vi "차선 보간(차량 가까운점).vi"(3 "Vision Theta":dbl[](array[numeric]), 4 "Vision Distance":dbl[](array[numeric]), 5 "Lane":dbl[][](array[numeric])) -> (0 "thetam":dbl[](array[numeric]), 1 "rm":dbl[](array[numeric]), 2 "Vision":dbl[][](array[numeric]))   [LabVIEW 2016]
uses:
  <vilib>/imath/engines/lvmath2/RunTimeEngine/Managers/WorkSpace/UID Generator.vi
  <vilib>/imath/engines/lvmath2/RunTimeEngine/RunTimeType/NIMS_RunTimeType_From StrictType (excl LVString).vi
  <instcachedir>/0/NIMS_RunTimeType_From StrictType (excl LVString)_BBF44FB49F834B71AF7A14CCEDF8BECD.lvgen/NIMS_RunTimeType_From StrictType (excl LVString)_BBF44FB49F834B71AF7A14CCEDF8BECD_000.vi
  <vilib>/imath/engines/lvmath2/RunTimeEngine/LocalVariableDefStatement/MC_LocalVariableDefStatement_Display.vi
  <vilib>/imath/engines/lvmath2/RunTimeEngine/MatrixToken/NIMS_MatrixToken_M_M.vi
  <instcachedir>/0/NIMS_MatrixToken_M_M_DF273B0CC20F424BBF1EDA9F4E71C841.lvgen/NIMS_MatrixToken_M_M_DF273B0CC20F424BBF1EDA9F4E71C841_003.vi
  <vilib>/imathl/engines/lvmath/Functions/Error Handling/Create Error.vi
  <vilib>/imath/engines/lvmath2/RunTimeEngine/Managers/SymbolTable/Clear UID.vi
  <vilib>/imath/engines/lvmath2/RunTimeEngine/NodeEndStatement/NIMS_NodeEndStatement_Output.vi
  <instcachedir>/0/NIMS_NodeEndStatement_Output_53EC0D466D134D7ABD903AC30B43404B.lvgen/NIMS_NodeEndStatement_Output_53EC0D466D134D7ABD903AC30B43404B_003.vi
  <instcachedir>/0/NIMS_NodeEndStatement_Output_53EC0D466D134D7ABD903AC30B43404B.lvgen/NIMS_NodeEndStatement_Output_53EC0D466D134D7ABD903AC30B43404B_000.vi
  <vilib>/imath/engines/lvmath2/RunTimeEngine/ErrorHandling/NIMS_Finalize Error.vi
  <vilib>/imath/engines/lvmath2/RunTimeEngine/Managers/SymbolTable/NIMS_WorkSpace.lvlib
panel:
  out "Xm":dbl[][](array[numeric])
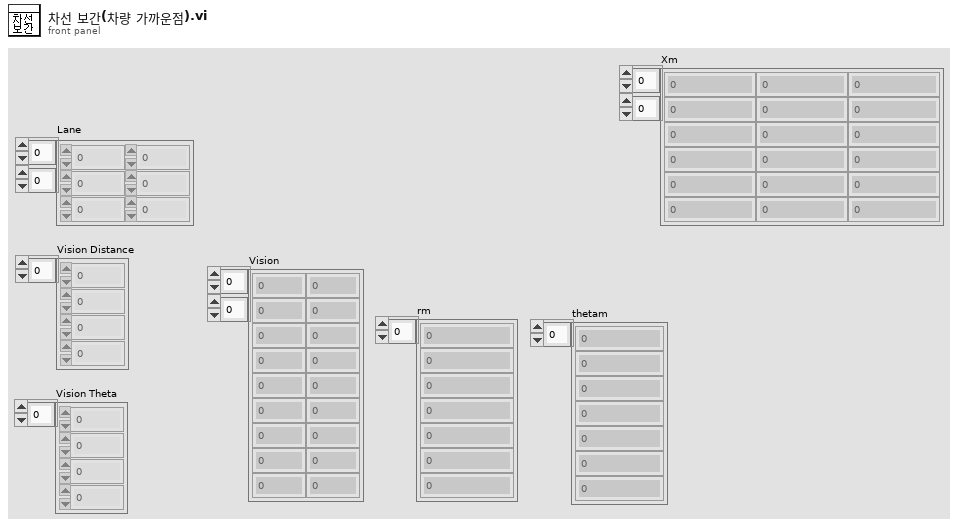
[diagram p1: front panel]
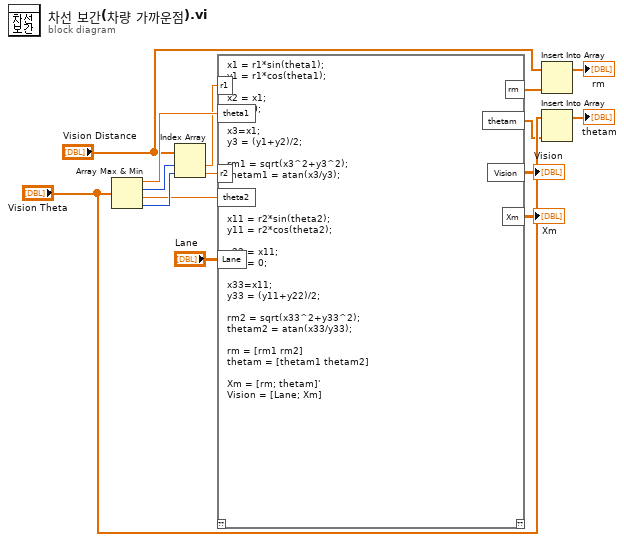
[diagram p0: block diagram]
diagram:
  n1 = Array Max & Min(array="Vision Theta") -> (max value=w13:dbl, max index (indices)=w15:i32, min value=w10:dbl, min index (indices)=w14:i32)
  n2 = Index Array(array="Vision Distance", index #1=w15, index #2=w14) -> (element #1=w12:dbl, element #2=w11:dbl)
  n3 = mathscript code="x1 = r1*sin(theta1);\ny1 = r1*cos(theta1);\n\nx2 = x1;\ny2 = 0;\n\nx3=x1;\ny3 = (y1+y2)/2;\n\nrm1 = sqrt(x3^2+y3^2);\nthetam1 = atan(x3/y3);\n\n\n\nx11 = r2*sin(theta2);\ny11 = r2*cos(theta2);\n\nx22 = x11;\ny22 = 0;\n\nx33=x11;\ny33 = (y11+y22)/2;\n\nrm2 = sqrt(x33^2+y33^2);\nthetam2 = atan(x33/y33);\n\nrm = [rm1 rm2]\nthetam = [thetam1 thetam2]\n\nXm = [rm; thetam]'\nVision = [Lane; Xm]"("r1"=w12, "theta1"=w13, "r2"=w11, "theta2"=w10, "Lane"="Lane") -> ("rm"=w8:cdb[], "thetam"=w6:cdb[], "Vision"=→"Vision":cdb[][], "Xm"=→"Xm":cdb[][])  [unwired: 1 in, 1 out]
  n4 = Insert Into Array(array="Vision Distance", new element=w8) -> (→"rm":dbl[])  [unwired: 1 in]
  n5 = Insert Into Array(array="Vision Theta", new element=w6) -> (→"thetam":dbl[])  [unwired: 1 in]
